vi "Simulate Error.vi"(8 "error in (no error)":errorcluster, 10 "Sim Error?":bool) -> (0 "error out":errorcluster)   [LabVIEW 2018]
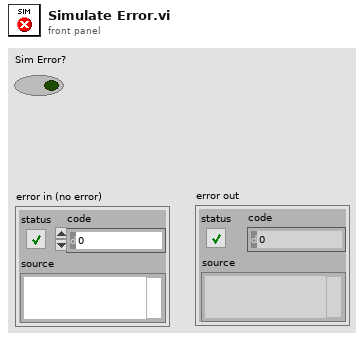
[diagram p1: front panel]
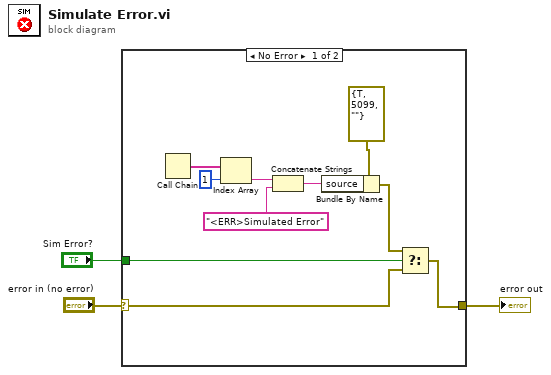
[diagram p0: block diagram]
diagram:
  n1 = case shown="No Error" "error in (no error)" {
    selector: "error in (no error)" -> [w5 w14]
    tunnel: "Sim Error?" -> [w7 _]
    tunnel: [w4 w14] -> w1
    frame No Error {
      n2 = Call Chain() -> (call chain=w13:string[])
      n3 = Index Array(array=w13, index=1) -> (element=w10:string)
      n4 = Concatenate Strings(w10, "<ERR>Simulated Error" ("string")) -> (w8:string)
      n5 = Bundle By Name(cluster=errorcluster {"status"=TRUE, "code"=5099, "source"=""} ("error in (no error)"), "source"=w8) -> (w6:errorcluster)
      n6 = Select(t=w6, s=w7, f=w5) -> (s? t:f=w4:errorcluster)
    }
    frame Error {
    }
  }
  "error out" <- w1
